vi "test CRUD job.vi"() -> ()   [LabVIEW 2019]
uses:
  <vilib>/httpClient/POSTBuffer.vi
  <vilib>/httpClient/LabVIEWHTTPClient.lvlib
panel:
  out "TABLE":string[][](table)
  out "body 2":string
  in  "JobId":string
  out "delete":string[](array[string])
  out "jobdesc":string[](array[string])
  out "jobno":string[](array[string])
  out "id":string[](array[string])
  out "status":string
  out "body":string
  in  "Job Description":string
  in  "Job No":string
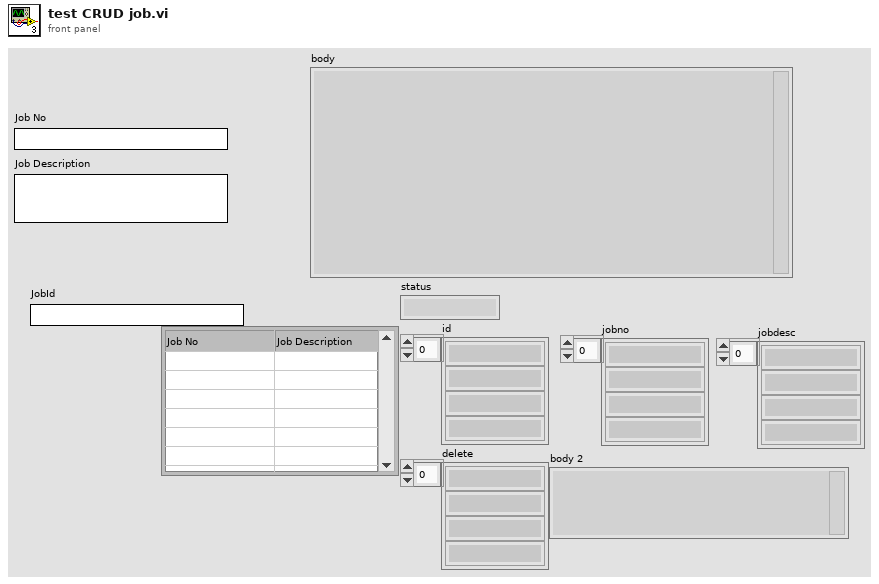
[diagram p1: front panel]
types:
  T1 = cluster{"action":string, "jobno":string, "jobdesc":string}
  T2 = cluster{"status":string, "data":cluster{"id":string, "jobno":string, "jobdesc":string, "delete":string}[]}
  T3 = typedef "LabVIEWHTTPClient.lvlib/ClientHandle.ctl" = refnum<k1>
  T4 = cluster{"id":string, "jobno":string, "jobdesc":string, "delete":string}[]
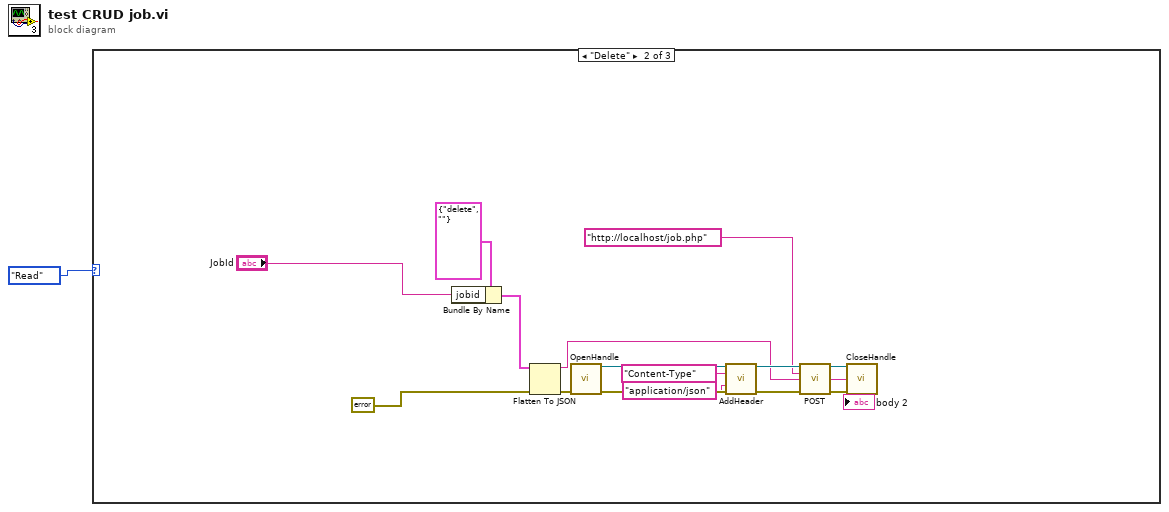
[diagram p0: block diagram]
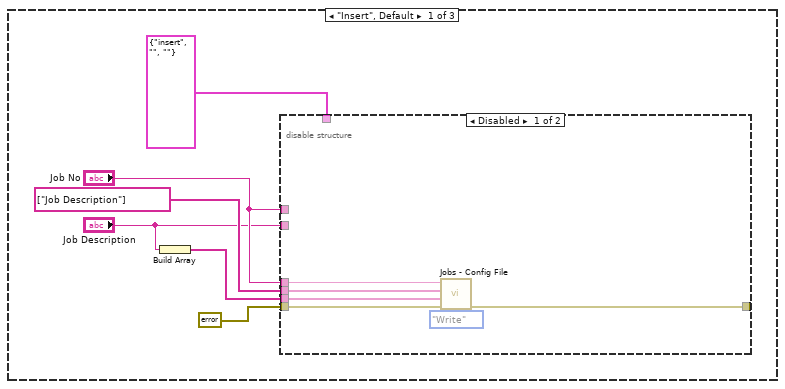
[diagram p2: hidden frame]
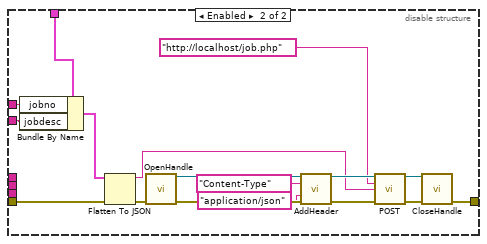
[diagram p3: hidden frame]
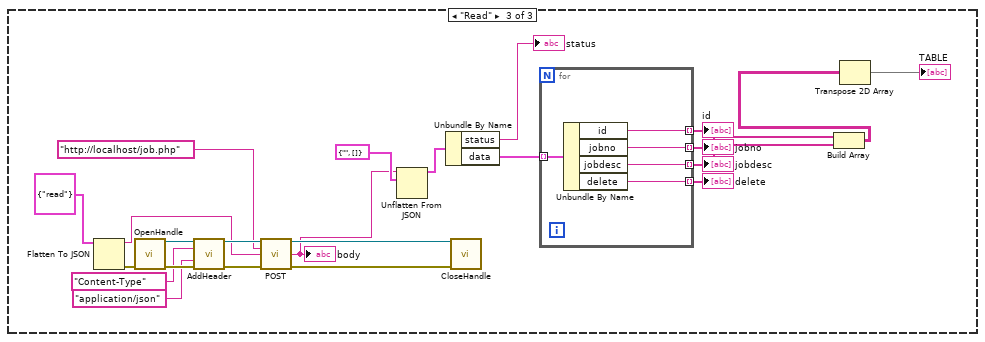
[diagram p4: hidden frame]
diagram:
  n1 = case shown="\"Delete\"" enum16{"Insert", "Read", "Delete"}."Read" {
    frame "Insert", Default {
      n2 = Build Array("Job Description") -> (w6:string[])
      n3 = disable-structure shown="Disabled" {
        disable-tunnel: errorcluster {"status"=FALSE, "code"=0, "source"=""} ("error IO") -> [w13 w14]
        disable-tunnel: [w12 w22] -> _
        disable-tunnel: "Job No" -> [w10 _]
        disable-tunnel: string[] ["Job Description"] ("Key Name") -> [w9 _]
        disable-tunnel: w6 -> [w8 _]
        disable-tunnel: T1 {"action"="insert", "jobno"="", "jobdesc"=""} -> [_ w19]
        disable-tunnel: "Job No" -> [_ w18]
        disable-tunnel: "Job Description" -> [_ w17]
        frame Disabled {
          n4 = call "Jobs - Config File.vi"("Action"=enum16{"Write", "Read", "Read All", "Remove"}."Write", "error in (no error)"=w13, "Value"=w8, "Key Name"=w9, "Jobs No"=w10) -> ("error out"=w12:errorcluster)  [unwired: 4 in, 2 out]
        }
        frame Enabled {
          n5 = Bundle By Name(cluster=w19, "jobno"=w18, "jobdesc"=w17) -> (w16:T1)
          n6 = Flatten To JSON(anything=w16, error in (no error)=w14) -> (JSON string=w15:string, 11:w20:errorcluster)  [unwired: 1 in]
          n7 = call <vilib>:"OpenHandle.vi"("error in (no error)"=w20) -> ("client handle out"=w28:T3, "error out"=w30:errorcluster)  [unwired: 13 in]
          n8 = call <vilib>:"AddHeader.vi"("client handle"=w28, "header"="Content-Type", "value"="application/json", "error in (no error)"=w30) -> ("client handle out"=w27:T3, "error out"=w29:errorcluster)  [unwired: 10 in]
          n9 = call-poly <vilib>:"POST.vi"("client handle"=w27, "url"="http://localhost/job.php", "buffer"=w15, "error in (no error)"=w29) -> ("client handle out"=w21:T3, "error out"=w23:errorcluster)  [unwired: 8 in, 2 out]
          n10 = call <vilib>:"CloseHandle.vi"("client handle"=w21, "error in (no error)"=w23) -> ("error out"=w22:errorcluster)  [unwired: 13 in]
        }
      }
    }
    frame "Delete" {
      n11 = Bundle By Name(cluster=cluster{"action":string, "jobid":string} {"action"="delete", "jobid"=""}, "jobid"="JobId") -> (w33:cluster{"action":string, "jobid":string})
      n12 = Flatten To JSON(anything=w33, error in (no error)=errorcluster {"status"=FALSE, "code"=0, "source"=""} ("error IO")) -> (JSON string=w32:string, 11:w34:errorcluster)  [unwired: 1 in]
      n13 = call <vilib>:"OpenHandle.vi"("error in (no error)"=w34) -> ("client handle out"=w41:T3, "error out"=w43:errorcluster)  [unwired: 13 in]
      n14 = call <vilib>:"AddHeader.vi"("client handle"=w41, "header"="Content-Type", "value"="application/json", "error in (no error)"=w43) -> ("client handle out"=w40:T3, "error out"=w42:errorcluster)  [unwired: 10 in]
      n15 = call-poly <vilib>:"POST.vi"("client handle"=w40, "url"="http://localhost/job.php", "buffer"=w32, "error in (no error)"=w42) -> ("client handle out"=w35:T3, "body"=→"body 2":string, "error out"=w36:errorcluster)  [unwired: 8 in, 1 out]
      n16 = call <vilib>:"CloseHandle.vi"("client handle"=w35, "error in (no error)"=w36) -> ()  [unwired: 13 in, 1 out]
    }
    frame "Read" {
      n17 = Flatten To JSON(anything=cluster{"action":string} {"action"="read"}) -> (JSON string=w62:string, 11:w63:errorcluster)  [unwired: 2 in]
      n18 = call <vilib>:"OpenHandle.vi"("error in (no error)"=w63) -> ("client handle out"=w67:T3, "error out"=w69:errorcluster)  [unwired: 13 in]
      n19 = call <vilib>:"AddHeader.vi"("client handle"=w67, "header"="Content-Type", "value"="application/json", "error in (no error)"=w69) -> ("client handle out"=w66:T3, "error out"=w68:errorcluster)  [unwired: 10 in]
      n20 = call-poly <vilib>:"POST.vi"("client handle"=w66, "url"="http://localhost/job.php", "buffer"=w62, "error in (no error)"=w68) -> ("client handle out"=w64:T3, "body"=w56:string, "error out"=w65:errorcluster)  [unwired: 8 in, 1 out]
      "body" <- w56
      n21 = Unflatten From JSON(JSON string=w56, type and defaults=T2 {"status"="", "data"=[]}) -> (value=w55:T2)  [unwired: 5 in, 1 out]
      n22 = Unbundle By Name(w55) -> ("status"=→"status":string, "data"=w54:T4)
      n23 = call <vilib>:"CloseHandle.vi"("client handle"=w64, "error in (no error)"=w65) -> ()  [unwired: 13 in, 1 out]
      n24 = for {
        tunnel: w54 -> [w74] mode=indexing
        tunnel: [w73] -> w52 mode=indexing
        tunnel: [w72] -> w50 mode=indexing
        tunnel: [w71] -> w49 mode=indexing
        tunnel: [w70] -> w51 mode=indexing
        n25 = Unbundle By Name(w74) -> ("id"=w73:string, "jobno"=w72:string, "jobdesc"=w71:string, "delete"=w70:string)
      }
      "id" <- w52
      "jobno" <- w50
      "jobdesc" <- w49
      "delete" <- w51
      n26 = Build Array(w50, w49) -> (w48:string[][])
      n27 = Transpose 2D Array(2D array=w48) -> (transposed array=→"TABLE":string[][])
    }
  }
